vi "Write.vi"(8 "error in (no error)":errorcluster, 10 "Characters to Write":string, 11 "VISA resource name in":refnum<visa-resource-name>) -> (0 "error out":errorcluster, 2 "Character Count":u32, 3 "VISA resource name out":refnum<visa-resource-name>)   [LabVIEW 2021, in "UART.lvlib"]
uses:
  <vilib>/myRIO/Instrument Drivers/Onboard IO/UART/UART.lvlib
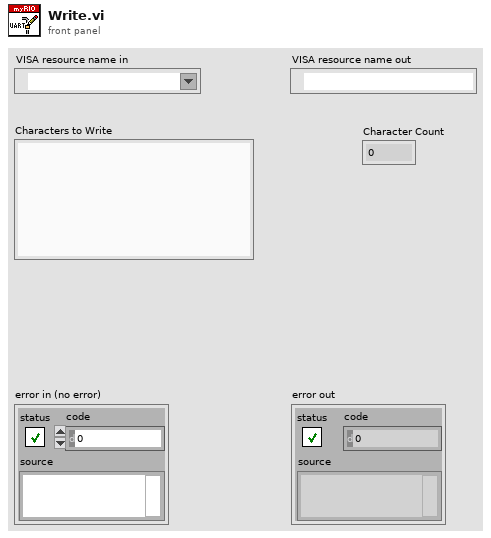
[diagram p1: front panel]
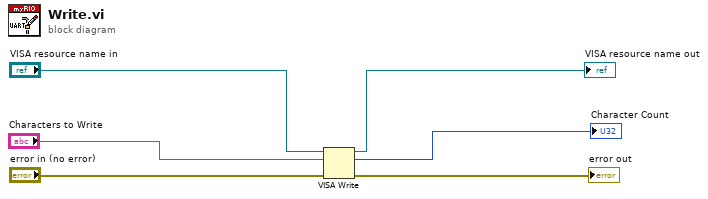
[diagram p0: block diagram]
diagram:
  n1 = VISA Write(VISA resource name="VISA resource name in", write buffer="Characters to Write", error in (no error)="error in (no error)") -> (VISA resource name out=→"VISA resource name out":refnum<visa-resource-name>, return count=→"Character Count":u32, error out=→"error out":errorcluster)
